vi "例3.7 提取当前VI的路径.vi"() -> ()   [LabVIEW 2017]
panel:
  out "最终路径":path
  out "拆分的路径":path
  out "当前VI的路径":path
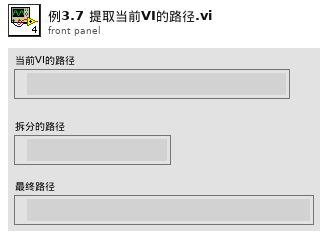
[diagram p1: front panel]
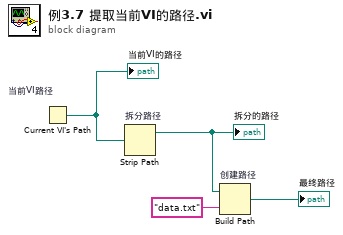
[diagram p0: block diagram]
diagram:
  n1 = Current VI's Path "当前VI路径"() -> (path=w4:path)
  "当前VI的路径" <- w4
  n2 = Strip Path "拆分路径"(path=w4) -> (stripped path=w1:path)  [unwired: 1 out]
  "拆分的路径" <- w1
  n3 = Build Path "创建路径"(base path=w1, name or relative path="data.txt" ("名称或相对路径")) -> (appended path=→"最终路径":path)
